vi "Refresh Statistics.vi"(6 "timeout (ms)":i32=5000, 8 "error in":errorcluster, 11 "gRPC ID":T1) -> (0 "error out":errorcluster, 3 "gRPC ID out":T1)   [LabVIEW 2021, in "CIFCoreWrapper.lvlib"]
uses:
  CIFCoreWrapper.lvlib
  <vilib>/gRPC/LabVIEW gRPC Library/Shared/grpcId.ctl
  CIFCorePlugin_client/CIFCorePlugin_client.lvlib
  <vilib>/gRPC/LabVIEW gRPC Library/grpc-lvsupport-release.lvlib
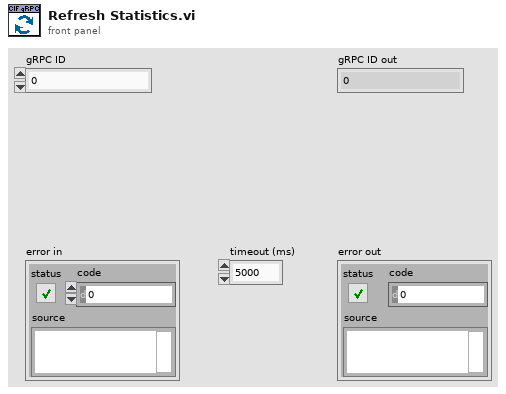
[diagram p1: front panel]
types:
  T1 = typedef "grpc-lvsupport-release.lvlib/grpcId.ctl" = u64
  T2 = typedef "CIFCorePlugin_client.lvlib/cif_plugincore_Status.ctl" = cluster{"code":i32, "message":string}
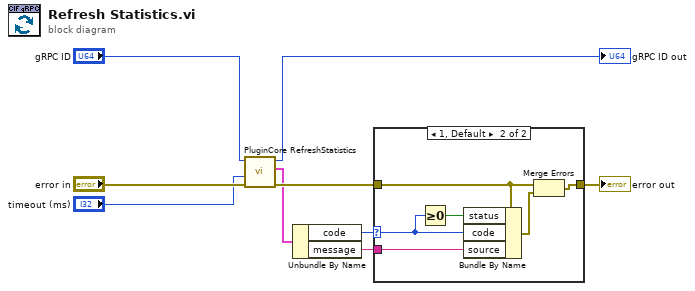
[diagram p0: block diagram]
diagram:
  n1 = call "PluginCore RefreshStatistics.vi"("error in"="error in", "timeout (ms)"="timeout (ms)", "gRPC ID"="gRPC ID") -> ("error out"=w4:errorcluster, "Response Data"=w1:T2, "gRPC ID out"=→"gRPC ID out":T1)  [unwired: 6 in]
  n2 = Unbundle By Name(w1) -> ("code"=w2:i32, "message"=w5:string)
  n3 = case shown="1, Default" w2 {
    selector: w2 -> [_ w11]
    tunnel: w5 -> [_ w15]
    tunnel: w4 -> [w10 w14]
    tunnel: [w10 w12] -> w3
    frame 0 {
    }
    frame 1, Default {
      n4 = Greater Or Equal To 0?(x=w11) -> (x >= 0?=w16:bool)
      n5 = Bundle By Name(cluster=w14, "status"=w16, "code"=w11, "source"=w15) -> (w13:errorcluster)
      n6 = Merge Errors(w14, w13) -> (w12:errorcluster)
    }
  }
  "error out" <- w3
